vi "Read offset of AC-DC element.vi"(8 "error in (no error)":errorcluster, 11 "FFmeter settings in":T1={"AC Source"={"AC Source type"=enum."Fluke 5XXX calibrator", "VISA"="", "Ref. clock (Hz)"=0.0, "status ref"=refnum}, "TWM pipe"="", "Measurement status ref"=refnum, "TWM Status ref"=refnum, "Abort ref"=refnum, "DC meter"={"DC meter type"=enum."H/A/K 3458", "DC meter VISA"="", "NPLC"=0, "No of readings"=3, "status ref"=refnum}, "Measurement properties"={"Measurement frequencies (Hz)"=[], "Sampling frequency (Hz)"=0.0, "Signal amplitude (V)"=0.0, "AC-DC settle time (s)"=20.0, "Record length (multiples of period)"=[1000.0, 10000.0, 1000.0], "Measurement template file"=path "", "Row of START keyword"=0, "Row of STOP keyword"=0, "Calculate RMS from samples"=FALSE}} {"Measurement properties"."Record length (multiples of period)" format="%#_3p"; "Measurement properties"."Sampling frequency (Hz)" format="%#_3p"; "Measurement properties"."Measurement frequencies (Hz)" format="%#_3p"}) -> (0 "error out":errorcluster, 2 "DC readings":dbl[](array[numeric]), 3 "FFmeter settings out":T1={"AC Source"={"AC Source type"=enum."Fluke 5XXX calibrator", "VISA"="", "Ref. clock (Hz)"=0.0, "status ref"=refnum}, "TWM pipe"="", "Measurement status ref"=refnum, "TWM Status ref"=refnum, "Abort ref"=refnum, "DC meter"={"DC meter type"=enum."H/A/K 3458", "DC meter VISA"="", "NPLC"=0, "No of readings"=3, "status ref"=refnum}, "Measurement properties"={"Measurement frequencies (Hz)"=[], "Sampling frequency (Hz)"=0.0, "Signal amplitude (V)"=0.0, "AC-DC settle time (s)"=20.0, "Record length (multiples of period)"=[1000.0, 10000.0, 1000.0], "Measurement template file"=path "", "Row of START keyword"=0, "Row of STOP keyword"=0, "Calculate RMS from samples"=FALSE}} {"Measurement properties"."Record length (multiples of period)" format="%#_3p"; "Measurement properties"."Sampling frequency (Hz)" format="%#_3p"; "Measurement properties"."Measurement frequencies (Hz)" format="%#_3p"})   [LabVIEW 2020]
uses:
  General AC source/Type definitions/AC Source type.ctl
  General AC source/Type definitions/AC Source.ctl
  General DC meter/Type definitions/DC meter type.ctl
  General DC meter/Type definitions/DC meter.ctl
  Type definitions/Measuement properties.ctl
  GUI/Type definitions/FFmeter settings.ctl
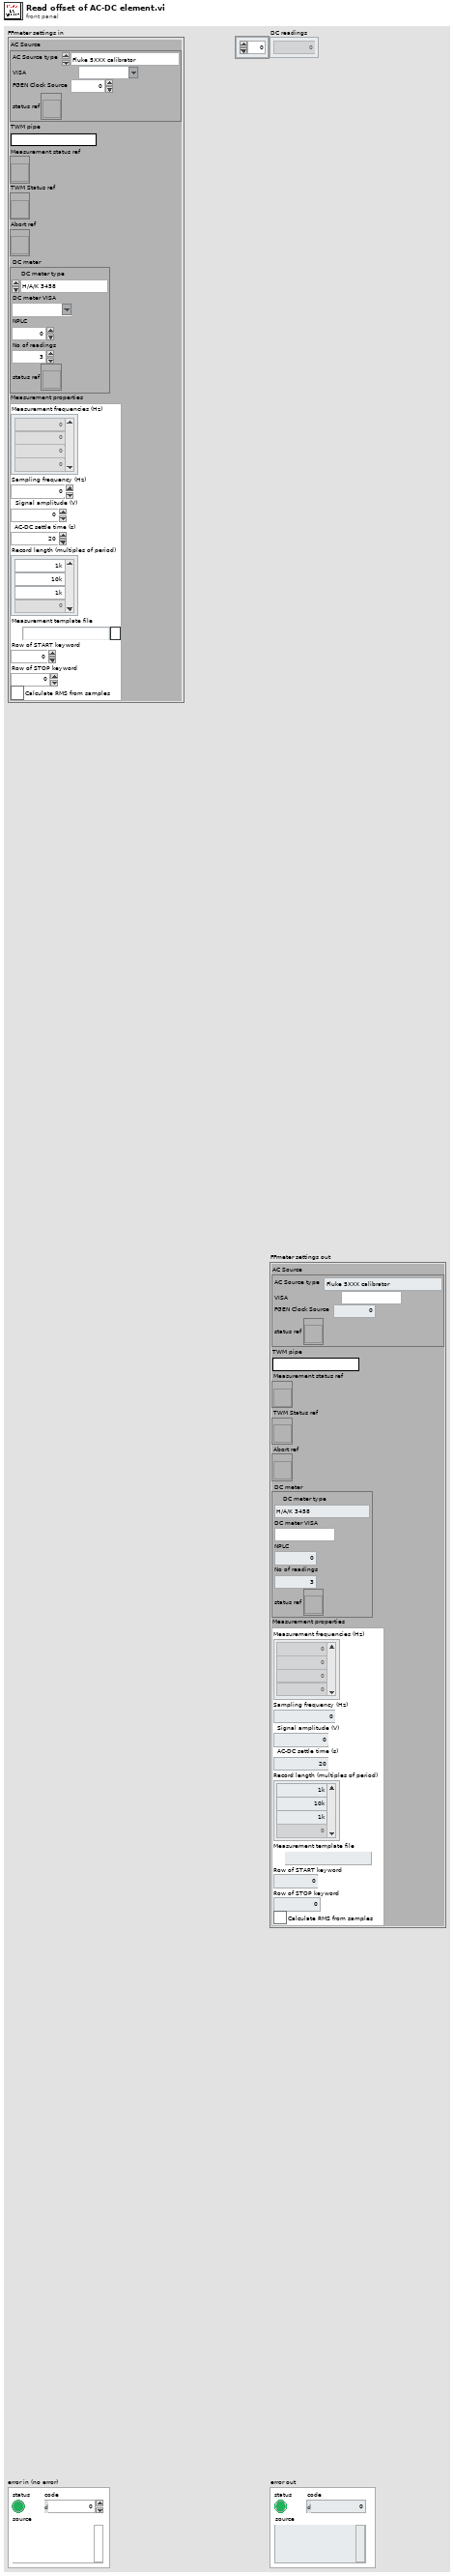
[diagram p1: front panel]
types:
  T1 = typedef "FFmeter settings.ctl" = cluster{"AC Source":T2, "TWM pipe":string, "Measurement status ref":refnum<vi>, "TWM Status ref":refnum<vi>, "Abort ref":refnum<vi>, "DC meter":T4, "Measurement properties":T6}
  T2 = typedef "AC Source.ctl" = cluster{"AC Source type":T3, "VISA":refnum<visa-resource-name>, "Ref. clock (Hz)":dbl, "status ref":refnum<vi>}
  T3 = typedef "AC Source type.ctl" = enum16{"Fluke 5XXX calibrator", "Tektronix AFG3101C", "dummy"}
  T4 = typedef "DC meter.ctl" = cluster{"DC meter type":T5, "DC meter VISA":refnum<visa-resource-name>, "NPLC":i32, "No of readings":i32, "status ref":refnum<vi>}
  T5 = typedef "DC meter type.ctl" = enum16{"H/A/K 3458", "FLuke 8508A", "dummy"}
  T6 = typedef "Measuement properties.ctl" = cluster{"Measurement frequencies (Hz)":dbl[], "Sampling frequency (Hz)":dbl, "Signal amplitude (V)":dbl, "AC-DC settle time (s)":dbl, "Record length (multiples of period)":dbl[], "Measurement template file":path, "Row of START keyword":i32, "Row of STOP keyword":i32, "Calculate RMS from samples":bool}
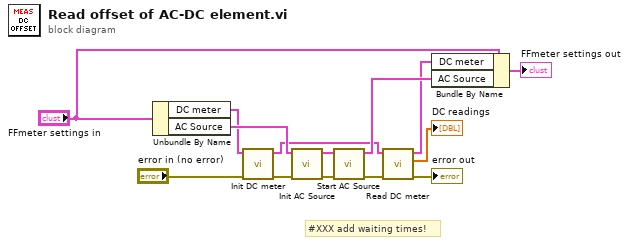
[diagram p0: block diagram]
diagram:
  # "#XXX add waiting times!"
  n1 = Unbundle By Name("FFmeter settings in") -> ("DC meter"=w6:T4, "AC Source"=w10:T2)
  n2 = call "Init DC meter.vi"("error in (no error)"="error in (no error)", "DC meter"=w6) -> ("error out"=w1:errorcluster, "DC meter out"=w9:T4)  [unwired: 7 in, 1 out]
  n3 = call "Init AC Source.vi"("error in (no error)"=w1, "AC source"=w10) -> ("error out"=w2:errorcluster, "AC source out"=w11:T2)  [unwired: 7 in, 1 out]
  n4 = call "Start AC Source.vi"("error in (no error)"=w2, "AC source"=w11) -> ("error out"=w3:errorcluster, "AC source out"=w12:T2)  [unwired: 7 in, 1 out]
  n5 = call "Read DC meter.vi"("error in (no error)"=w3, "DC meter"=w9) -> ("error out"=→"error out":errorcluster, "DC readings"=→"DC readings":dbl[], "DC meter out"=w8:T4)  [unwired: 7 in]
  n6 = Bundle By Name(cluster="FFmeter settings in", "DC meter"=w8, "AC Source"=w12) -> (→"FFmeter settings out":T1)
